vi "Close Digital Session.vi"(7 "pin list":string, 8 "error in":errorcluster, 11 "Digital session":refnum<k15>) -> (0 "error out":errorcluster)   [LabVIEW 2021]
uses:
  <instrlib>/niDigital/niDigital.llb/niDigital Selected Function.ctl
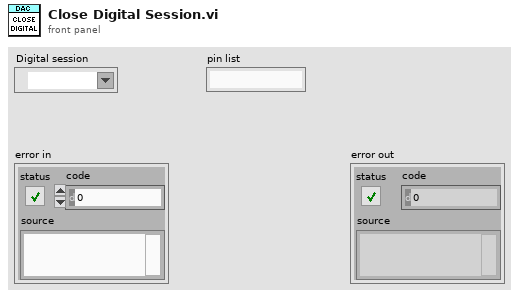
[diagram p1: front panel]
types:
  T1 = typedef "niDigital Selected Function.ctl" = i32
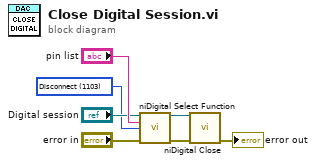
[diagram p0: block diagram]
diagram:
  w4 = T1 1103 items=["Digital"=1100, "PPMU"=1101, "Off"=1102, "Disconnect"=1103] ("function")
  n1 = call <instrlib>:"niDigital Select Function.vi"("instrument handle"="Digital session", "channel list"="pin list", "function"=w4, "error in"="error in") -> ("instrument handle out"=w2:refnum<k15>, "error out"=w3:errorcluster)  [unwired: 10 in]
  n2 = call <instrlib>:"niDigital Close.vi"("instrument handle"=w2, "error in"=w3) -> ("error out"=→"error out":errorcluster)  [unwired: 13 in]
